vi "openeod.vi"(0 "Byte Stream File in":refnum<file>, 1 "size (in bytes)":i64, 5 "error in (no error)":errorcluster) -> (6 "Wave":i16[][](array[numeric]), 8 "nchar":u8[](array[numeric]), 9 "polarity":i8[](array[numeric]), 10 "nWavepoints":u32[](array[numeric]), 11 "userdata":sgl[][](array[numeric]), 12 "Numeric":i32, 13 "nbytes":i8[](array[numeric]), 14 "Byte Stream File out":refnum<file>, 15 "ADrange":sgl[](array[numeric]), 16 "eodtext":string[](array[string]), 17 "srate":u32[](array[numeric]), 18 "nbits":i8[](array[numeric]), 19 "error out":errorcluster)   [LabVIEW 2012]
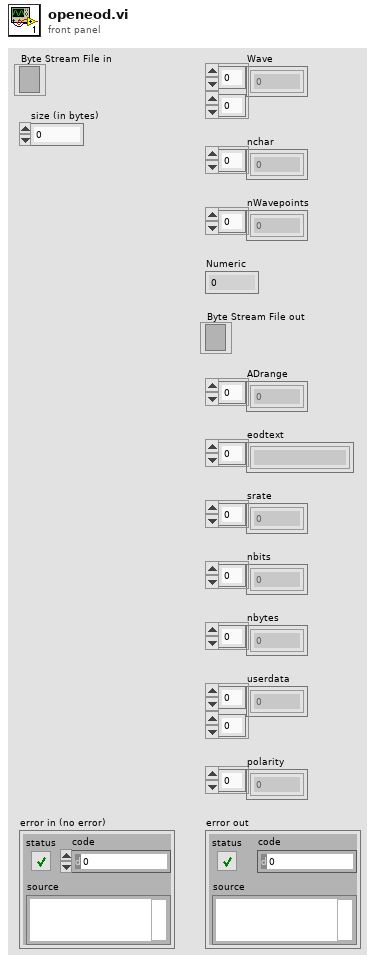
[diagram p1: front panel]
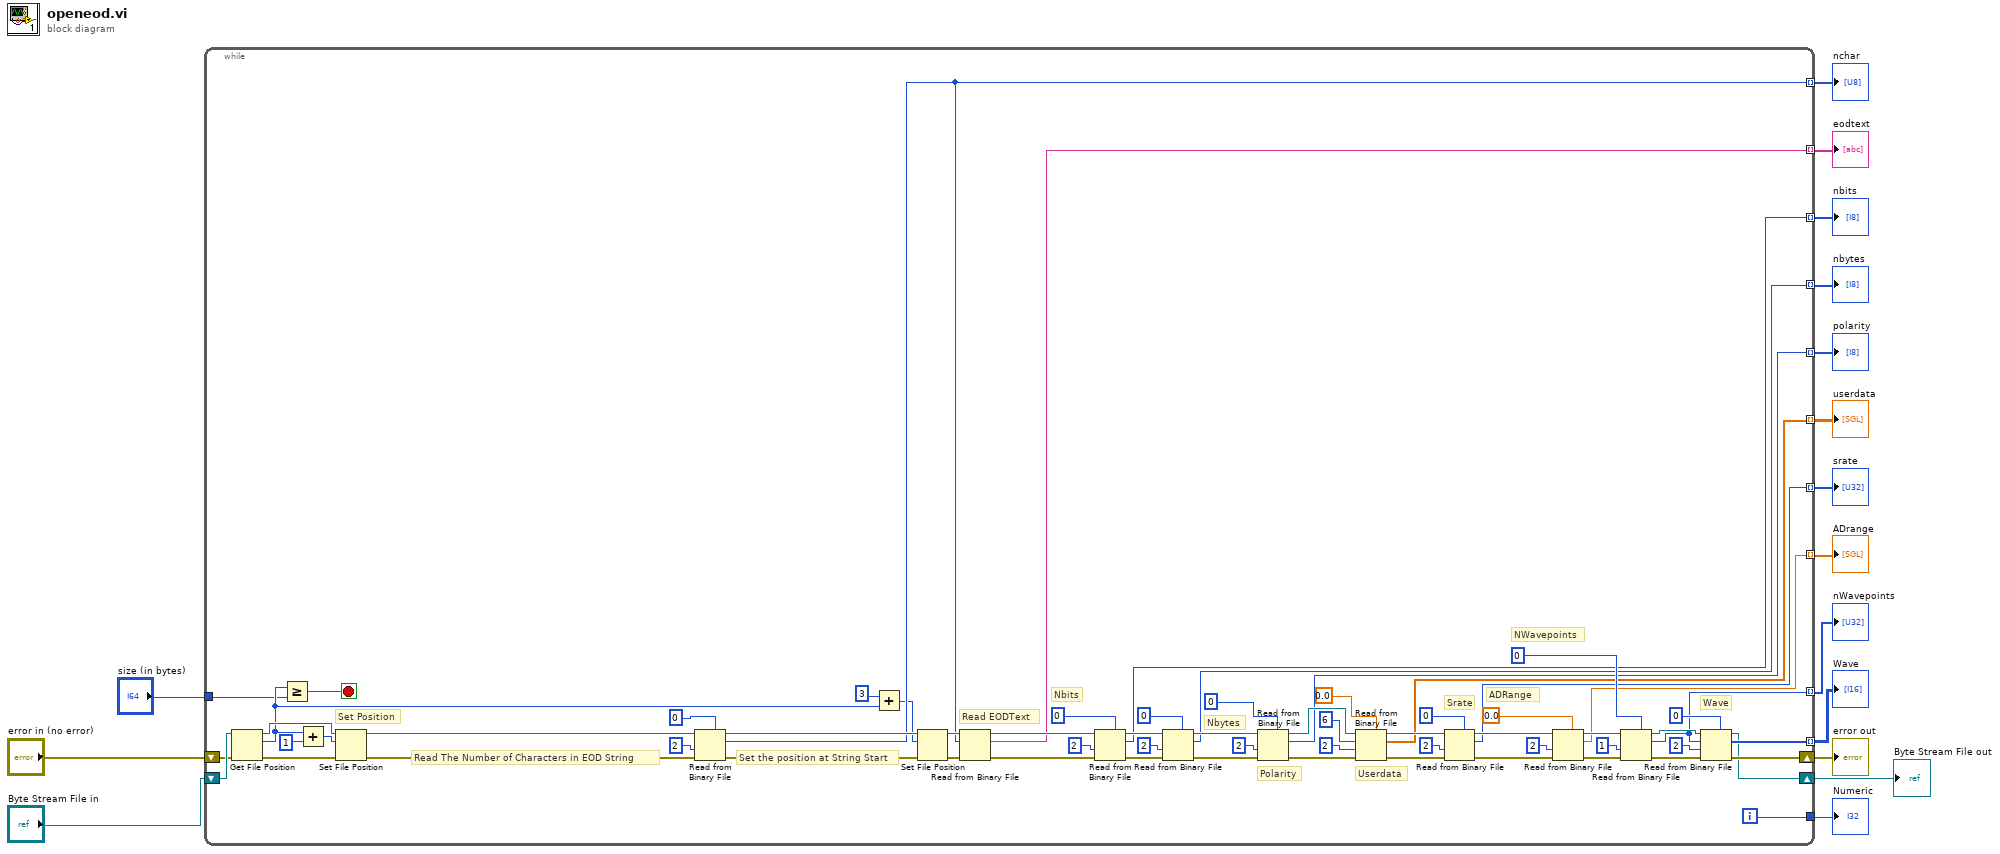
[diagram p0: block diagram]
diagram:
  n1 = while {
    tunnel: [w51] -> w1 mode=indexing
    tunnel: [w50] -> w2 mode=indexing
    tunnel: [w49] -> w3 mode=indexing
    tunnel: [w48] -> w4 mode=indexing
    tunnel: [w47] -> w5 mode=indexing
    tunnel: [w46] -> w6 mode=indexing
    tunnel: [w45] -> w7 mode=indexing
    tunnel: [w44] -> w8 mode=indexing
    tunnel: [w43] -> w10 mode=indexing
    tunnel: [w42] -> w9 mode=indexing
    shift-right: [w18] -> w14
    shift-left: "Byte Stream File in" -> [w29]
    shift-right: [w25] -> w15
    shift-left: "error in (no error)" -> [w26]
    tunnel: "size (in bytes)" -> [w19]
    tunnel: [w17] -> w13
    i -> [w17]
    stop <- w30 stop-if-true
    # "Wave"
    # "NWavepoints"
    # "ADRange"
    # "Srate"
    # "Userdata"
    # "Polarity"
    # "Nbytes"
    # "Nbits"
    # "Read EODText"
    # "Set the position at String Start"
    # "Read The Number of Characters in EOD String"
    # "Set Position"
    n2 = Get File Position(4:w26, 7:w29) -> (0:w27:errorcluster, 2:w20:i64, 3:w28:refnum<file>)
    n3 = Greater Or Equal?(x=w20, y=w19) -> (x >= y?=w30:bool)
    n4 = Add(x=w20, y=1) -> (x+y=w23:i64)
    n5 = Set File Position(offset (in bytes) (0)=w23, refnum=w28, error in=w27) -> (refnum out=w80:refnum<file>, error out=w41:errorcluster)  [unwired: 1 in]
    n6 = Read from Binary File(5:u8 0, 8:w41, 9:2, 11:w80) -> (0:w40:errorcluster, 2:w51:u8, 3:w79:refnum<file>)  [unwired: 2 in, 1 out]
    n7 = Add(x=3, y=w20) -> (x+y=w22:i64)
    n8 = Set File Position(offset (in bytes) (0)=w22, refnum=w79, error in=w40) -> (refnum out=w78:refnum<file>, error out=w39:errorcluster)  [unwired: 1 in]
    n9 = Read from Binary File(8:w39, 10:w51, 11:w78) -> (0:w38:errorcluster, 2:w50:string, 3:w77:refnum<file>)  [unwired: 3 in, 1 out]
    n10 = Read from Binary File(5:i8 0, 8:w38, 9:2, 11:w77) -> (0:w37:errorcluster, 2:w49:i8, 3:w53:refnum<file>)  [unwired: 2 in, 1 out]
    n11 = Read from Binary File(5:i8 0, 8:w37, 9:2, 11:w53) -> (0:w36:errorcluster, 2:w48:i8, 3:w54:refnum<file>)  [unwired: 2 in, 1 out]
    n12 = Read from Binary File(5:i8 0, 8:w36, 9:2, 11:w54) -> (0:w35:errorcluster, 2:w47:i8, 3:w52:refnum<file>)  [unwired: 2 in, 1 out]
    n13 = Read from Binary File(5:sgl 0.0, 8:w35, 9:2, 10:6, 11:w52) -> (0:w34:errorcluster, 2:w46:sgl[], 3:w74:refnum<file>)  [unwired: 1 in, 1 out]
    n14 = Read from Binary File(5:u32 0, 8:w34, 9:2, 11:w74) -> (0:w33:errorcluster, 2:w45:u32, 3:w66:refnum<file>)  [unwired: 2 in, 1 out]
    n15 = Read from Binary File(5:sgl 0.0, 8:w33, 9:2, 11:w66) -> (0:w32:errorcluster, 2:w44:sgl, 3:w60:refnum<file>)  [unwired: 2 in, 1 out]
    n16 = Read from Binary File(5:u32 0, 8:w32, 9:1, 11:w60) -> (0:w31:errorcluster, 2:w42:u32, 3:w61:refnum<file>)  [unwired: 2 in, 1 out]
    n17 = Read from Binary File(5:i16 0, 8:w31, 9:2, 10:w42, 11:w61) -> (0:w25:errorcluster, 2:w43:i16[], 3:w18:refnum<file>)  [unwired: 1 in, 1 out]
  }
  "error out" <- w15
  "Byte Stream File out" <- w14
  "Numeric" <- w13
  "Wave" <- w10
  "nWavepoints" <- w9
  "ADrange" <- w8
  "srate" <- w7
  "userdata" <- w6
  "polarity" <- w5
  "nbytes" <- w4
  "nbits" <- w3
  "eodtext" <- w2
  "nchar" <- w1
